vi "close_data_file.vi"(8 "error in":errorcluster, 10 "Final integral":dbl, 11 "file refnum in":refnum<file>) -> (0 "error out":errorcluster, 3 "file refnum outs":refnum<file>)   [LabVIEW 2010]
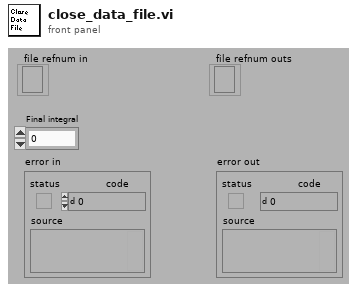
[diagram p1: front panel]
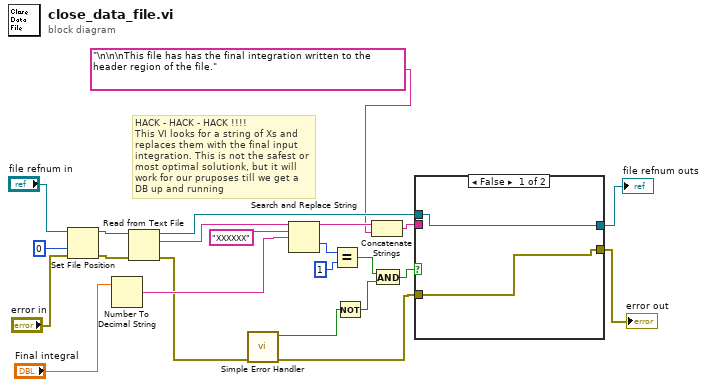
[diagram p0: block diagram]
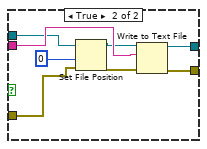
[diagram p2: hidden frame]
diagram:
  # "HACK - HACK - HACK !!!! \nThis VI looks for a string of Xs and replaces them with the final input integration. This is not the safest or most optimal solutionk, but it will work for our pruposes till we get a DB up and running"
  n1 = Set File Position(refnum="file refnum in", from (0:start)=0, error in="error in") -> (refnum out=w20:refnum<file>, error out=w19:errorcluster)  [unwired: 1 in]
  n2 = Number To Decimal String(number="Final integral") -> (decimal integer string=w15:string)  [unwired: 1 in]
  n3 = Read from Text File(file (use dialog)=w20, error in=w19) -> (refnum out=w6:refnum<file>, text=w18:string, error out=w11:errorcluster)  [unwired: 2 in, 1 out]
  n4 = call <vilib>:"Simple Error Handler.vi"("error in (no error)"=w11) -> ("error?"=w8:bool, "error out"=w5:errorcluster)  [unwired: 4 in, 3 out]
  n5 = Search and Replace String(input string=w18, search string="XXXXXX", replace string=w15) -> (result string=w14:string, offset past replacement=w13:i32)  [unwired: 5 in, 2 out]
  n6 = Equal?(x=w13, y=1) -> (x = y?=w10:bool)
  n7 = Not(x=w8) -> (.not. x?=w7:bool)
  n8 = Concatenate Strings(w14, "\n\n\nThis file has has the final integration written to the header region of the file.") -> (w4:string)
  n9 = And(x=w10, y=w7) -> (x .and. y?=w9:bool)
  n10 = case shown="False" w9 {
    tunnel: w4 -> [_ w33]
    tunnel: w6 -> [w24 w32]
    tunnel: w5 -> [w25 w31]
    tunnel: [w24 w27] -> w2
    tunnel: [w25 w26] -> w1
    frame False {
    }
    frame True {
      n11 = Set File Position(refnum=w32, from (0:start)=0, error in=w31) -> (refnum out=w29:refnum<file>, error out=w30:errorcluster)  [unwired: 1 in]
      n12 = Write to Text File(file (use dialog)=w29, text=w33, error in=w30) -> (refnum out=w27:refnum<file>, error out=w26:errorcluster)  [unwired: 1 in, 1 out]
    }
  }
  "file refnum outs" <- w2
  "error out" <- w1
